vi "Get Nested Enq.vi"(8 "error in":errorcluster, 10 "Ident":string, 11 "Series Actor in":refnum<class "Series Actor.lvclass">) -> (0 "error out":errorcluster, 1 "Enq":refnum<class "Message Enqueuer.lvclass">, 3 "Series Actor out":refnum<class "Series Actor.lvclass">)   [LabVIEW 2024, in "Series Actor.lvlib" / "Series Actor.lvclass"]
uses:
  Series Actor.lvclass
  Series Actor.lvclass/Series Actor.ctl
  <vilib>/ActorFramework/Message Enqueuer/Message Enqueuer.lvclass
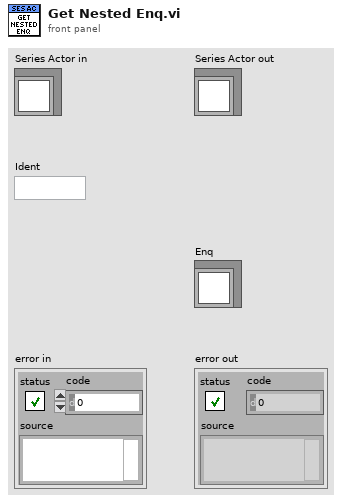
[diagram p1: front panel]
types:
  T1 = map{string, refnum<class "Message Enqueuer.lvclass">}
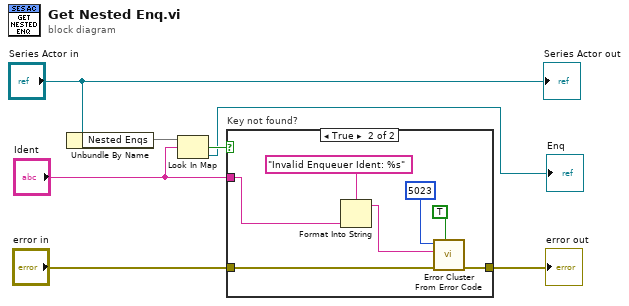
[diagram p0: block diagram]
diagram:
  n1 = Unbundle By Name("Series Actor in") -> ("Nested Enqs"=w6:T1)
  n2 = Look In Map(map=w6, key="Ident") -> (key not found?=w5:bool, value=→"Enq":refnum<class "Message Enqueuer.lvclass">)  [unwired: 1 in]
  n3 = case "Key not found?" shown="True" w5 {
    tunnel: "error in" -> [w8 w15]
    tunnel: [w8 w12] -> w3
    tunnel: "Ident" -> [_ w10]
    frame False {
    }
    frame True {
      n4 = Format Into String(format string="Invalid Enqueuer Ident: %s", w10) -> (resulting string=w9:string)  [unwired: 2 in, 1 out]
      n5 = call <vilib>:"Error Cluster From Error Code.vi"("show call chain? (False)"=TRUE, "error in (no error)"=w15, "error message (\"\")"=w9, "error code (0)"=5023) -> ("error out"=w12:errorcluster)  [unwired: 5 in]
    }
  }
  "error out" <- w3
  "Series Actor out" <- "Series Actor in"
